vi "PathPlanner_Trajectory_New.vi"(8 "Reversed":bool, 9 "MaxAccel":dbl, 10 "MaxVelocity":dbl, 11 "PathPoints":T1[](array[typedef]) {"HolonomicRotation"."SIN" format="%13.4f"; "HolonomicRotation"."COS" format="%13.4f"; "HolonomicRotation"."VALUE" format="%13.4f"; "NextControl"."Y" format="%14.3f"; "NextControl"."X" format="%14.3f"; "PrevControl"."Y" format="%14.3f"; "PrevControl"."X" format="%14.3f"; "AnchorPoint"."Y" format="%14.3f"; "AnchorPoint"."X" format="%14.3f"}) -> (3 "PathPlannerTrajectory":T4 {"States"."TargetHolonomicRotation"."SIN" format="%13.4f"; "States"."TargetHolonomicRotation"."COS" format="%13.4f"; "States"."TargetHolonomicRotation"."VALUE" format="%13.4f"; "States"."Heading"."SIN" format="%13.4f"; "States"."Heading"."COS" format="%13.4f"; "States"."Heading"."VALUE" format="%13.4f"; "States"."PositionMeters"."Y" format="%14.3f"; "States"."PositionMeters"."X" format="%14.3f"})   [LabVIEW 2019, in "PathPlanner24.lvlib"]
uses:
  PathPlanner24.lvlib
  <vilib>/Rock Robotics/WPI/ThirdParty/JAS_Junk/TrajLib/TypeDef/ROTATION2D.ctl
  <vilib>/Rock Robotics/WPI/ThirdParty/JAS_Junk/TrajLib/Trajectory_Library.lvlib
  <vilib>/Rock Robotics/WPI/ThirdParty/JAS_Junk/TrajLib/TypeDef/TRANSLATION2D.ctl
  PathPlannerTrajectoryState.ctl
  PathPlannerTrajectory.ctl
  PathPlannerConstraints.ctl
  PathPlannerWaypoint.ctl
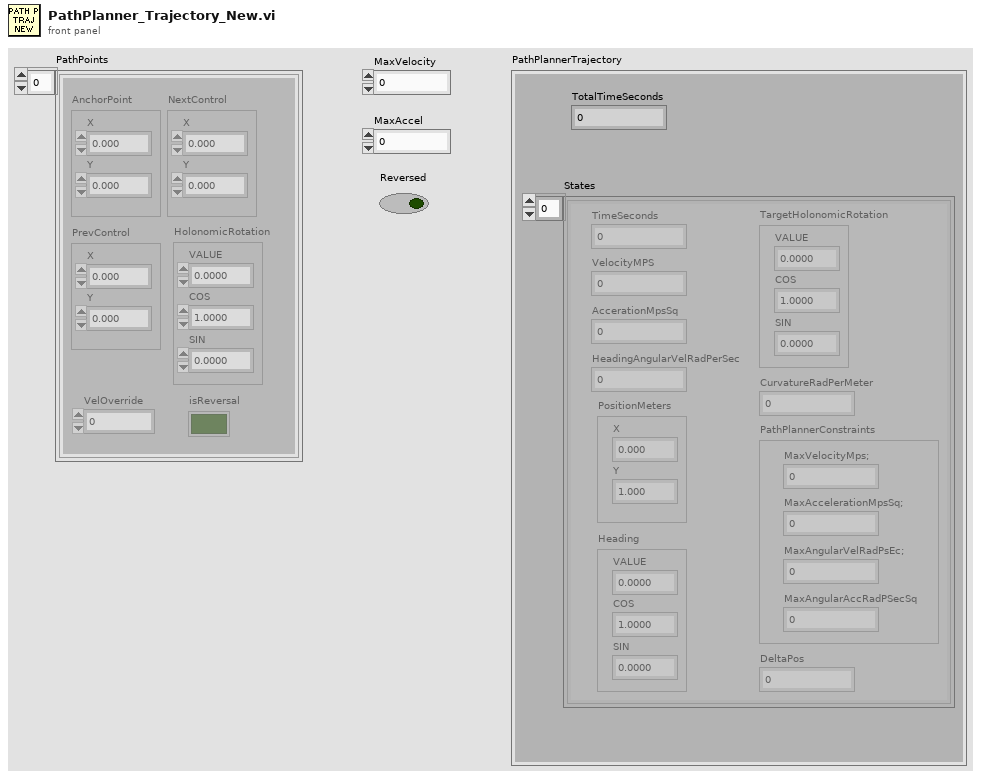
[diagram p1: front panel]
types:
  T1 = typedef "PathPlanner24.lvlib/PathPlannerWaypoint.ctl" = cluster{"AnchorPoint":T2, "PrevControl":T2, "NextControl":T2, "HolonomicRotation":T3, "VelOverride":dbl, "isReversal":bool}
  T2 = typedef "Trajectory_Library.lvlib/TRANSLATION2D.ctl" = cluster{"X":dbl, "Y":dbl}
  T3 = typedef "Trajectory_Library.lvlib/ROTATION2D.ctl" = cluster{"VALUE":dbl, "COS":dbl, "SIN":dbl}
  T4 = typedef "PathPlanner24.lvlib/PathPlannerTrajectory.ctl" = cluster{"TotalTimeSeconds":dbl, "States":T5[]}
  T5 = typedef "PathPlanner24.lvlib/PathPlannerTrajectoryState.ctl" = cluster{"TimeSeconds":dbl, "VelocityMPS":dbl, "AccerationMpsSq":dbl, "HeadingAngularVelRadPerSec":dbl, "PositionMeters":T2, "Heading":T3, "TargetHolonomicRotation":T3, "CurvatureRadPerMeter":dbl, "DeltaPos":dbl, "PathPlannerConstraints":T6}
  T6 = typedef "PathPlanner24.lvlib/PathPlannerConstraints.ctl" = cluster{"MaxVelocityMps;":dbl, "MaxAccelerationMpsSq;":dbl, "MaxAngularVelRadPsEc;":dbl, "MaxAngularAccRadPSecSq":dbl}
  T7 = typedef "PathPlanner24.lvlib/PathPlannerTrajectory.ctl" = cluster{"States":T5[]}
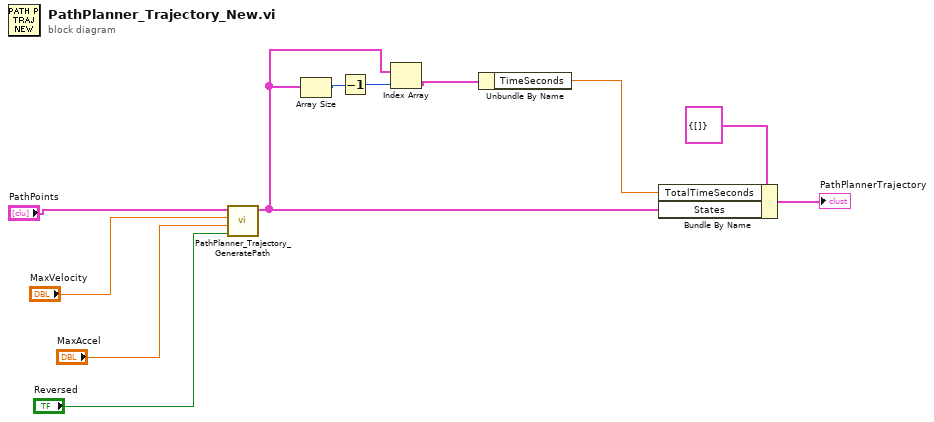
[diagram p0: block diagram]
diagram:
  n1 = call "PathPlanner_Trajectory_GeneratePath.vi"("Reversed"="Reversed", "MaxAccel"="MaxAccel", "MaxVel"="MaxVelocity", "PathPoints"="PathPoints") -> ("PathPlannerStates"=w3:T5[])  [unwired: 7 in]
  n2 = Array Size(array=w3) -> (size(s)=w4:i32)
  n3 = Decrement(x=w4) -> (x-1=w5:i32)
  n4 = Index Array(array=w3, index=w5) -> (element=w2:T5)
  n5 = Unbundle By Name(w2) -> ("TimeSeconds"=w1:dbl)
  n6 = Bundle By Name(cluster=T7 {"States"=[]} ("PathPlannerTrajectory"), "TotalTimeSeconds"=w1, "States"=w3) -> (→"PathPlannerTrajectory":T7)
